vi "VPA QC Final Checklist.vi"(7 "DAQ Q":T3, 9 "DAQ Ref Cluster":T1, 10 "State Cluster":T4) -> (2 "State Cluster Out":T4)   [LabVIEW 2013]
uses:
  Controls/VPA QC State Data Cluster.ctl
  Controls/VPA QC General Cluster.ctl
  Controls/VPA QC State Enum.ctl
  Controls/VPA QC Bool Cluster.ctl
  Controls/VPA QC DAQ Q.ctl
  Controls/VPA QC DAQ Cmd Enum.ctl
  Controls/VPA QC DAQ Ref Cluster.ctl
  Controls/VPA QC Scale Communication Settings DVR.ctl
  Controls/VPA QC Scale Communication Settings.ctl
  <userlib>/_MGI/Timing/MGI Wait/MGI Wait (U32).vi
panel:
  in  "Clean Water Out":bool caption="Take off the manifold and clear all water out of the cylinders and manifold"
  in  "Maintenance Hours":bool caption="Reset Maintenance hours from the initial setup menu."
  in  "Initialize Pump":bool caption="Initilaize pump to get the cylinders to top position."
  in  "Wrap":bool caption="Wrap pump in plastic visqueen."
  out "DAQ Err":bool
  in  "Cancel":bool
  in  "Ok":bool
  in  "Burn":bool caption="Burn new calibration constants to memory."
  in  "Box":bool caption="Place VPA in box and all other required parts"
  in  "Screws":bool caption="Verify that all screws are tight"
  in  "Covers":bool caption="Install remaining covers"
  in  "Check Fact Rest":bool caption="Go to factory settings and then verify that new constants are still in program"
  # "Final Checklist"
  # "Assembly Checklist"
  # "Assembly Checklist"
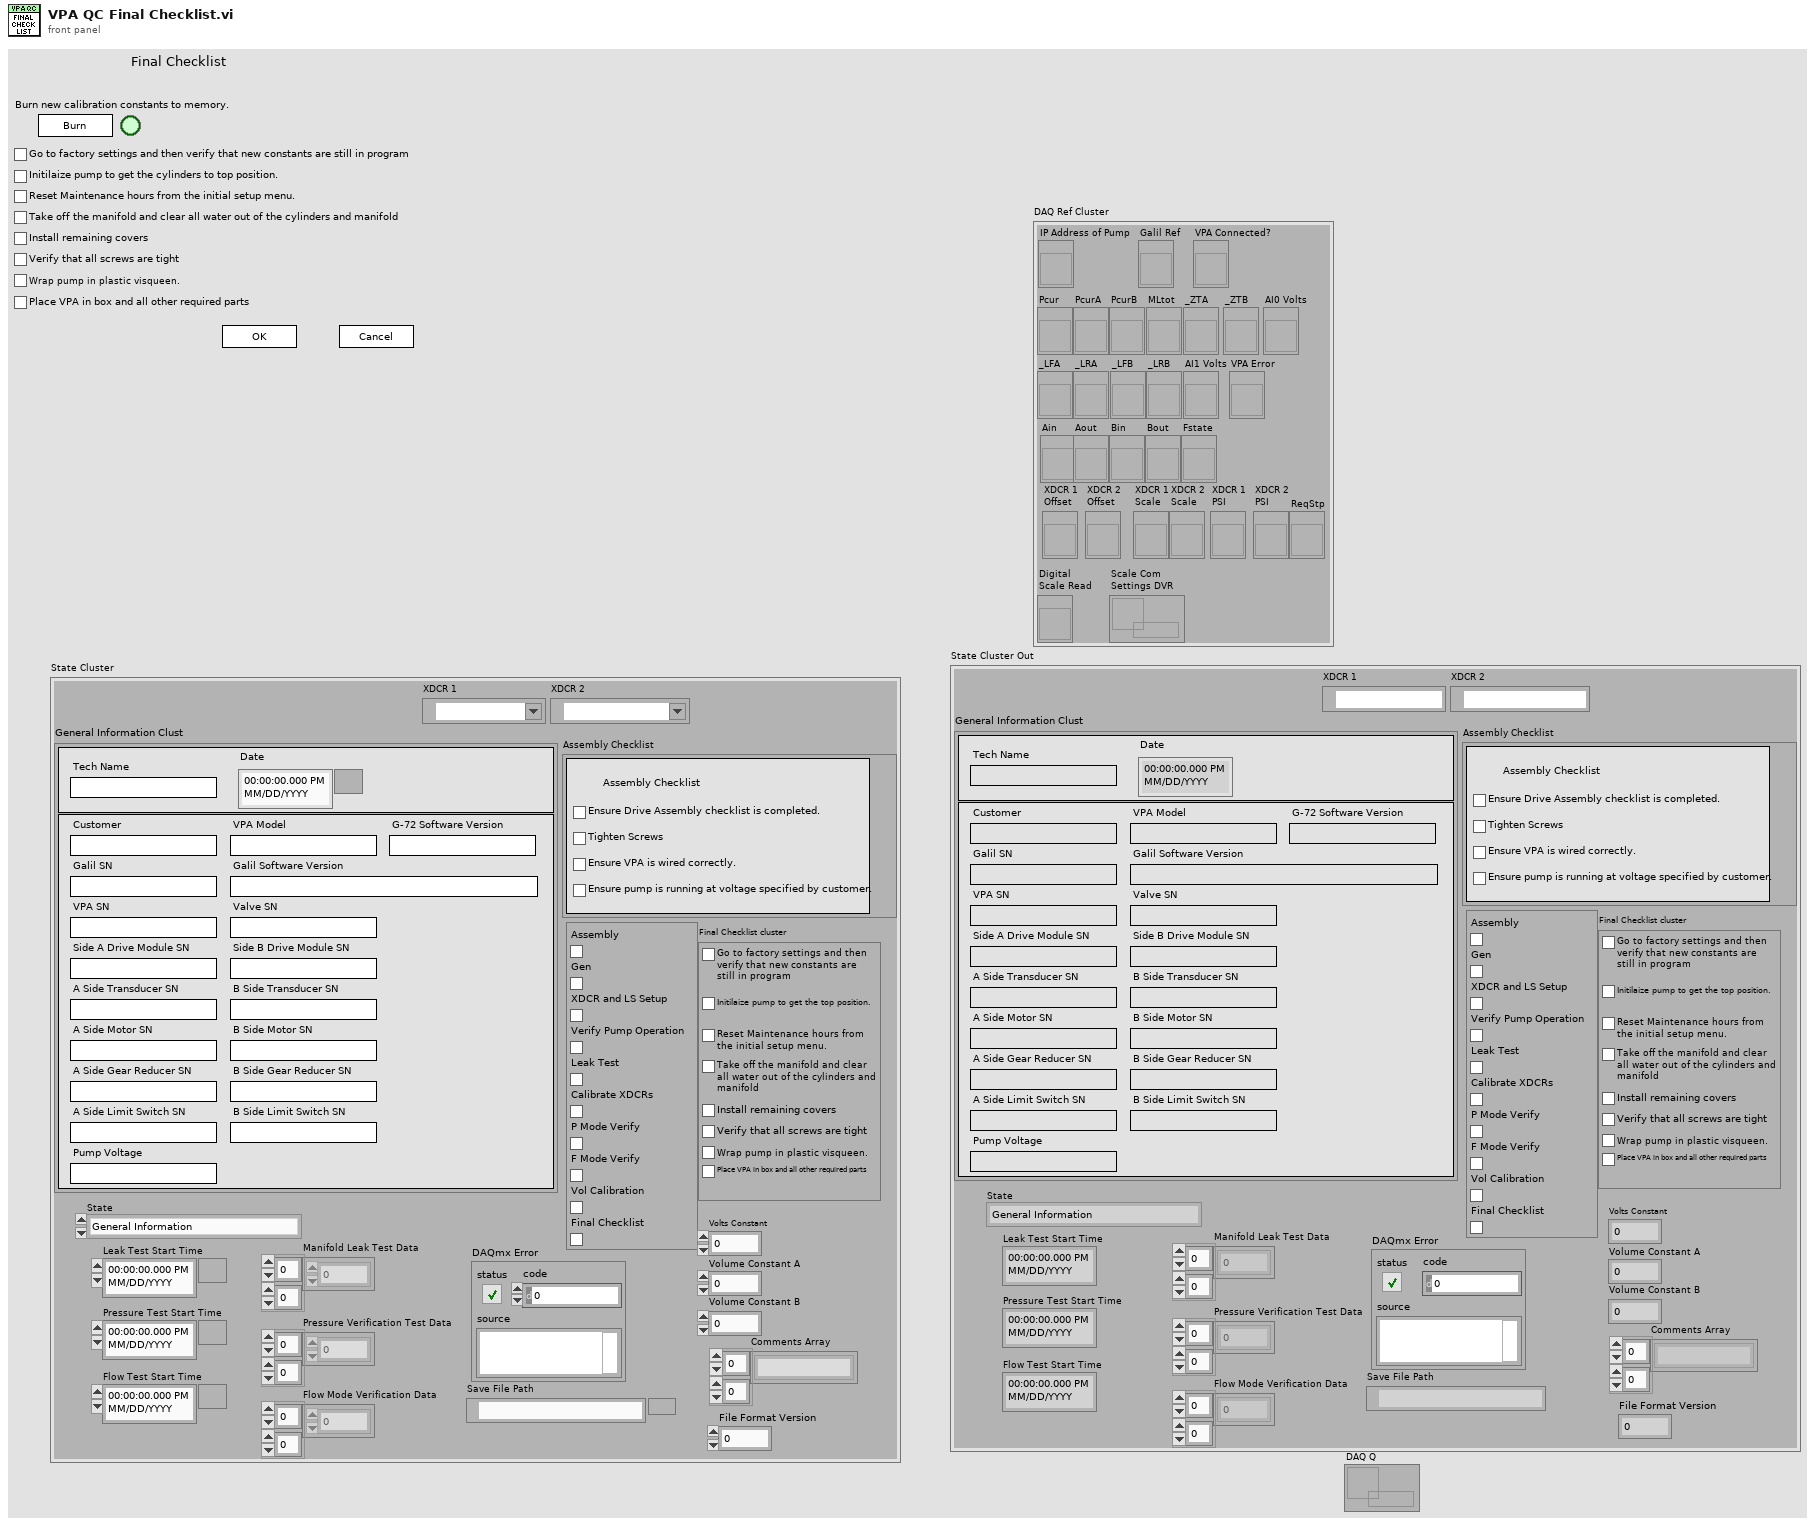
[diagram p1: front panel]
types:
  T1 = typedef "VPA QC DAQ Ref Cluster.ctl" = cluster{"IP Address of Pump":refnum<vi>, "Galil Ref":refnum<vi>, "VPA Connected?":refnum<vi>, "Pcur":refnum<vi>, "PcurA":refnum<vi>, "PcurB":refnum<vi>, "MLtot":refnum<vi>, "_LFA":refnum<vi>, "_LRA":refnum<vi>, "_LFB":refnum<vi>, "_LRB":refnum<vi>, "_ZTA":refnum<vi>, "_ZTB":refnum<vi>, "AI0 Volts":refnum<vi>, "AI1 Volts":refnum<vi>, "VPA Error":refnum<vi>, "Ain":refnum<vi>, "Aout":refnum<vi>, "Bin":refnum<vi>, "Bout":refnum<vi>, "Fstate":refnum<vi>, "XDCR 1\nOffset":refnum<vi>, "XDCR 2 \nOffset":refnum<vi>, "XDCR 1\nScale":refnum<vi>, "XDCR 2\nScale":refnum<vi>, "XDCR 1\nPSI":refnum<vi>, "XDCR 2\nPSI":refnum<vi>, "ReqStp":refnum<vi>, "Digital \nScale Read":refnum<vi>, "Scale Com\nSettings DVR":T2}
  T2 = typedef "VPA QC Scale Communication Settings DVR.ctl" = refnum<data-value>
  T3 = typedef "VPA QC DAQ Q.ctl" = refnum<queue>
  T4 = typedef "VPA QC State Data Cluster.ctl" = cluster{"XDCR 1":tag, "XDCR 2":tag, "General Information Clust":T5, "Assembly Checklist":cluster{"Ensure Drive Assembly checklist is completed.":bool, "Tighten Screws":bool, "Ensure VPA is wired correctly.":bool, "Ensure pump is running at voltage specified by customer.":bool}, "State":T6, "Manifold Leak Test Data":dbl[][], "Pressure Verification Test Data":dbl[][], "Flow Mode Verification Data":dbl[][], "DAQmx Error":errorcluster, "Bool Cluster":T7, "Leak Test Start Time":timestamp, "Pressure Test Start Time":timestamp, "Flow Test Start Time":timestamp, "Final Checklist cluster":cluster{"Check Fact Rest":bool, "Initialize Pump":bool, "Maintenance Hours":bool, "Clean Water Out":bool, "Covers":bool, "Screws":bool, "Wrap":bool, "Box":bool}, "Volts Constant":dbl, "Volume Constant A":dbl, "Volume Constant B":dbl, "Save File Path":path, "Comments Array":string[][], "File Format Version":u16}
  T5 = typedef "VPA QC General Cluster.ctl" = cluster{"Tech Name":string, "Date":timestamp, "Customer":string, "VPA Model":string, "G-72 Software Version":string, "Galil SN":string, "Galil Software Version":string, "VPA SN":string, "Valve SN":string, "Side A Drive Module SN":string, "Side B Drive Module SN":string, "A Side Transducer SN":string, "B Side Transducer SN":string, "A Side Motor SN":string, "B Side Motor SN":string, "A Side Gear Reducer SN":string, "B Side Gear Reducer SN":string, "A Side Limit Switch SN":string, "B Side Limit Switch SN":string, "Pump Voltage":string}
  T6 = typedef "VPA QC State Enum.ctl" = enum16{"General Information", "XDCR and LS Check", "Check Pump Function", "Manifold/Cylinder Leak Test", "Exit"}
  T7 = typedef "VPA QC Bool Cluster.ctl" = cluster{"Assembly":bool, "Gen":bool, "XDCR and LS Setup":bool, "Verify Pump Operation":bool, "Leak Test":bool, "Calibrate XDCRs":bool, "P Mode Verify":bool, "F Mode Verify":bool, "Vol Calibration":bool, "Final Checklist":bool}
  T8 = typedef "VPA QC DAQ Cmd Enum.ctl" = enum16{"Connect", "Disconnect", "Quit", "Close All Valves", "Burn Calibration", "E-Stop", "Set ZC1", "Set ZC0", "Set ZR", "Open Outlet Valves"}
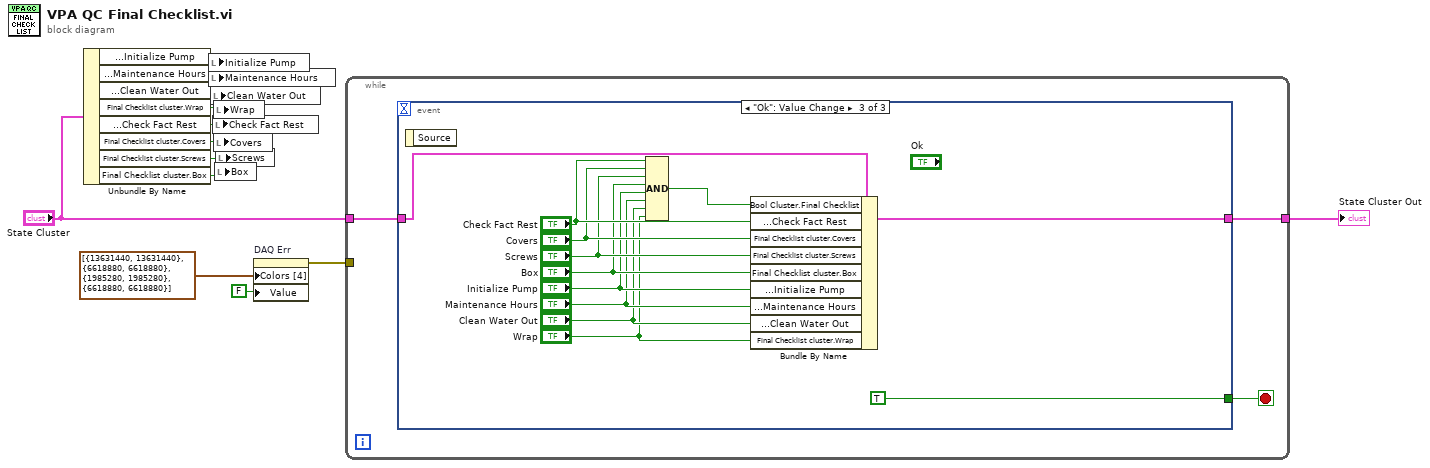
[diagram p0: block diagram]
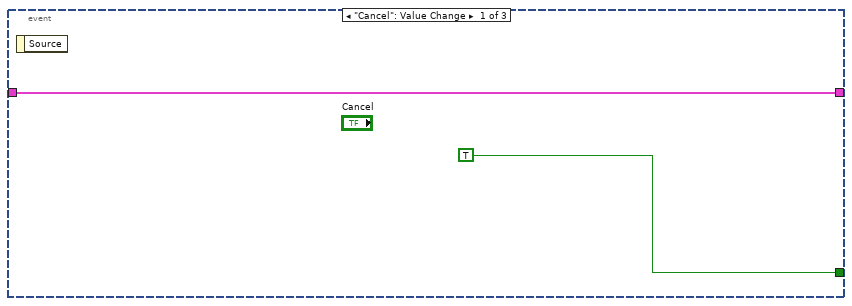
[diagram p2: hidden frame]
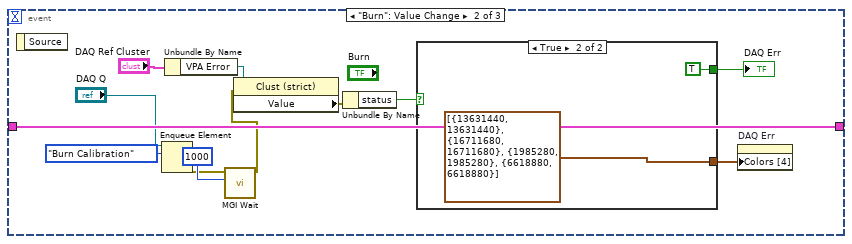
[diagram p3: hidden frame]
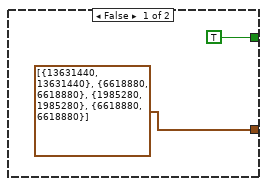
[diagram p4: hidden frame]
diagram:
  n1 = Unbundle By Name("State Cluster") -> ("Final Checklist cluster.Initialize Pump"=w2:bool, "Final Checklist cluster.Maintenance Hours"=w4:bool, "Final Checklist cluster.Clean Water Out"=w1:bool, "Final Checklist cluster.Wrap"=w3:bool, "Final Checklist cluster.Check Fact Rest"=w11:bool, "Final Checklist cluster.Covers"=w10:bool, "Final Checklist cluster.Screws"=w9:bool, "Final Checklist cluster.Box"=w8:bool)
  n2 = local write "Initialize Pump"(w2) -> ()
  n3 = local write "Maintenance Hours"(w4) -> ()
  n4 = local write "Clean Water Out"(w1) -> ()
  n5 = local write "Check Fact Rest"(w11) -> ()
  n6 = local write "Wrap"(w3) -> ()
  n7 = local write "Covers"(w10) -> ()
  n8 = local write "Box"(w8) -> ()
  n9 = local write "Screws"(w9) -> ()
  n10 = property on="DAQ Err" class="Bool (strict)"("Colors [4]"=cluster{u32, u32}[] [{13631440, 13631440}, {6618880, 6618880}, {1985280, 1985280}, {6618880, 6618880}], "Value"=FALSE ("DAQ Err")) -> (error out=w6:errorcluster)  [unwired: 2 in, 1 out]
  n11 = while {
    tunnel: "State Cluster" -> [w15]
    tunnel: [w14] -> w13
    tunnel: w6 -> [_]
    stop <- w16 stop-if-true
    n12 = event shown="[2] \"Ok\": Value Change" {
      selector: _ -> [_ _ _]
      dyn-events: _ -> [_ _ _]
      timeout: _ -> [_ _ _]
      tunnel: [TRUE _ TRUE] -> w16
      tunnel: w15 -> [w17 w30 w45]
      tunnel: [w17 w30 w44] -> w14
      event "Cancel": Value Change {
        n13 = event-data() -> ()  [unwired: 1 in, 1 out]
      }
      event "Burn": Value Change {
        n14 = event-data() -> ()  [unwired: 1 in, 1 out]
        n15 = Enqueue Element(queue="DAQ Q", element=VPA_QC_DAQ_Cmd_Enum."Burn Calibration") -> (error out=w22:errorcluster)  [unwired: 2 in, 2 out]
        n16 = Unbundle By Name("DAQ Ref Cluster") -> ("VPA Error"=w26:refnum<vi>)
        n17 = call-poly <userlib>:"MGI Wait.vi"("ms"=u32 1000, "Error In"=w22) -> ("Error Out"=w23:errorcluster)  [unwired: 5 in]
        n18 = property class="Clust (strict)"(reference=w26, error in=w23) -> ("Value"=w25:errorcluster)  [unwired: 2 out]
        n19 = Unbundle By Name(w25) -> ("status"=w20:bool)
        n20 = case shown="True" w20 {
          tunnel: [cluster{u32, u32}[] [{13631440, 13631440}, {6618880, 6618880}, {1985280, 1985280}, {6618880, 6618880}] ("Colors [4]") cluster{u32, u32}[] [{13631440, 13631440}, {16711680, 16711680}, {1985280, 1985280}, {6618880, 6618880}] ("Colors [4]")] -> w21
          tunnel: [TRUE ("DAQ Err") TRUE ("DAQ Err")] -> w19
          frame False {
          }
          frame True {
          }
        }
        "DAQ Err" <- w19
        n21 = property on="DAQ Err" class="Bool (strict)"("Colors [4]"=w21) -> ()  [unwired: 2 in, 2 out]
      }
      event "Ok": Value Change {
        n22 = event-data() -> ()  [unwired: 1 in, 1 out]
        n23 = Compound Arithmetic op=AND("Check Fact Rest", "Covers", "Screws", "Box", "Initialize Pump", "Maintenance Hours", "Clean Water Out", "Wrap") -> (w39:bool)
        n24 = Bundle By Name(cluster=w45, "Bool Cluster.Final Checklist"=w39, "Final Checklist cluster.Check Fact Rest"="Check Fact Rest", "Final Checklist cluster.Covers"="Covers", "Final Checklist cluster.Screws"="Screws", "Final Checklist cluster.Box"="Box", "Final Checklist cluster.Initialize Pump"="Initialize Pump", "Final Checklist cluster.Maintenance Hours"="Maintenance Hours", "Final Checklist cluster.Clean Water Out"="Clean Water Out", "Final Checklist cluster.Wrap"="Wrap") -> (w44:T4)
      }
    }
  }
  "State Cluster Out" <- w13
